vi "Add.vi"(8 "error in (no error)":errorcluster, 10 "Data1D 2":refnum<class "Data1D.lvclass">, 11 "Data1D in":refnum<class "Data1D.lvclass">) -> (0 "error out":errorcluster, 3 "Data1D out":refnum<class "Data1D.lvclass">)   [LabVIEW 2014, in "Data1D.lvclass"]
uses:
  Data1D.lvclass
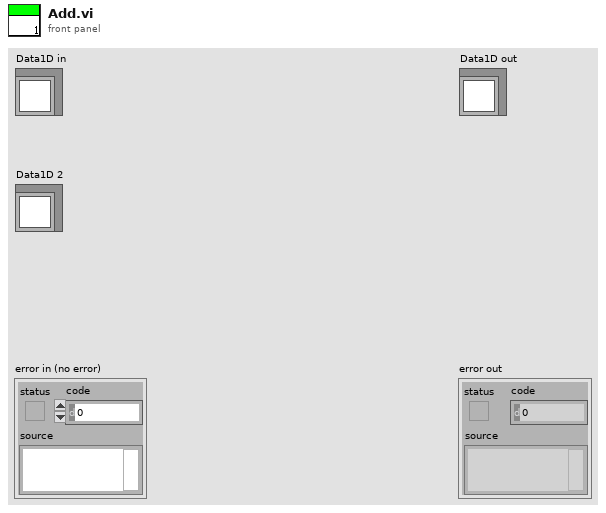
[diagram p1: front panel]
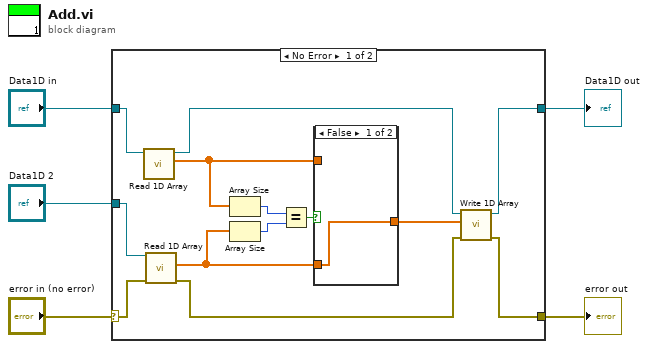
[diagram p0: block diagram]
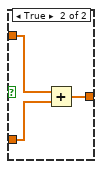
[diagram p2: hidden frame]
diagram:
  n1 = case shown="No Error" "error in (no error)" {
    selector: "error in (no error)" -> [w11 w24]
    tunnel: [w6 w24] -> w4
    tunnel: [w15 w23] -> w2
    tunnel: "Data1D in" -> [w9 w23]
    tunnel: "Data1D 2" -> [w13 _]
    frame No Error {
      n2 = call "Read 1D Array.vi"("Data1D in"=w9) -> ("1D Array"=w10:dbl[], "Data1D out"=w8:refnum<class "Data1D.lvclass">)  [unwired: 8 in, 1 out]
      n3 = call "Read 1D Array.vi"("error in (no error)"=w11, "Data1D in"=w13) -> ("error out"=w7:errorcluster, "1D Array"=w12:dbl[])  [unwired: 7 in, 1 out]
      n4 = Array Size(array=w10) -> (size(s)=w17:i32)
      n5 = Array Size(array=w12) -> (size(s)=w18:i32)
      n6 = Equal?(x=w17, y=w18) -> (x = y?=w16:bool)
      n7 = case shown="False" w16 {
        tunnel: w10 -> [_ w22]
        tunnel: w12 -> [w19 w21]
        tunnel: [w19 w20] -> w14
        frame False {
        }
        frame True {
          n8 = Add(x=w22, y=w21) -> (x+y=w20:dbl[])
        }
      }
      n9 = call "Write 1D Array.vi"("error in (no error)"=w7, "1D Array"=w14, "Data1D in"=w8) -> ("error out"=w6:errorcluster, "Data1D out"=w15:refnum<class "Data1D.lvclass">)  [unwired: 7 in]
    }
    frame Error {
    }
  }
  "error out" <- w4
  "Data1D out" <- w2
